vi "RSZVB Add Limit Line Segment.vi"(0 "VISA session":refnum<visa-resource-name>, 1 "Stop Stimulus (0.0)":dbl format="%^.3e", 2 "Stop Response (0.0)":dbl format="%^.3e", 5 "Channel (Trace) (1)":i32=1, 7 "Segment (1)":i32=1, 9 "Type (1: Upper)":i32(ring)=1 items=["Off", "Upper", "Lower"], 11 "error in (no error)":errorcluster {"code" format="%.0x"}, 12 "Start Response (0.0)":dbl format="%^.3e", 13 "Start Stimulus (0.0)":dbl format="%^.3e") -> (4 "dup VISA session":refnum<visa-resource-name>, 15 "error out":errorcluster {"code" format="%.0x"})   [LabVIEW 2011]
doc: "This VI adds a new segment to the limit line list. In each segment the limit line is defined as a straight line connecting two points.\n\nNote(s):\n\nThis VI does not overwrite existing limit line segments. The defined segment is appended to the segment list as new segment.\n\nRemote-control command(s):\nCALCulate<Ch/Tr>:LIMit:DATA <type>, <start_stim>, <stop_stim>, <start_resp>, <stop_resp>"
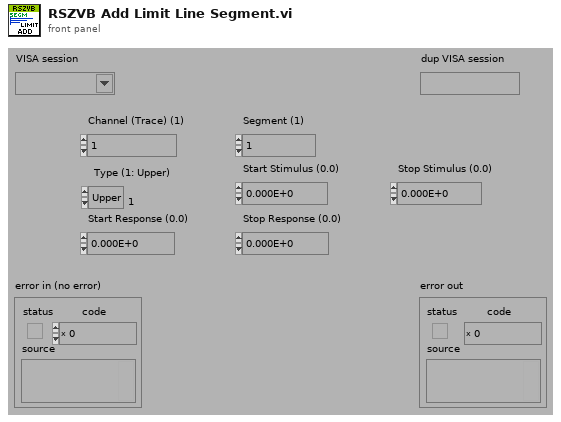
[diagram p1: front panel]
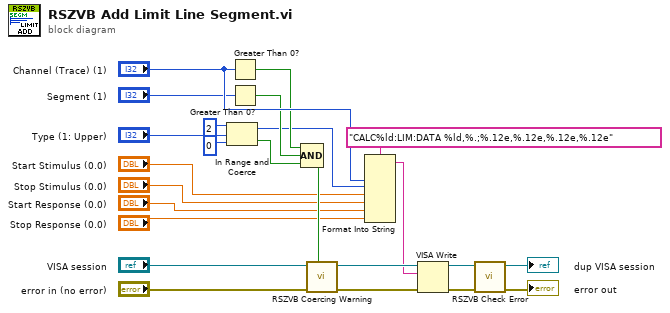
[diagram p0: block diagram]
diagram:
  n1 = In Range and Coerce(upper limit=2, x="Type (1: Upper)", lower limit=0) -> (coerced(x)=w2:i32, In Range?=w17:bool)
  n2 = Greater Than 0?(x="Channel (Trace) (1)") -> (x > 0?=w4:bool)
  n3 = Greater Than 0?(x="Segment (1)") -> (x > 0?=w3:bool)
  n4 = Compound Arithmetic op=AND(w4, w3, w17) -> (w16:bool)
  n5 = call "RSZVB Coercing Warning.vi"("In Range?"=w16, "error in (no error)"="error in (no error)", "VISA session"="VISA session") -> ("error out"=w23:errorcluster, "dup VISA session"=w24:refnum<visa-resource-name>)  [unwired: 7 in]
  n6 = Format Into String(format string="CALC%ld:LIM:DATA %ld,%.;%.12e,%.12e,%.12e,%.12e", "Channel (Trace) (1)", w2, "Start Stimulus (0.0)", "Stop Stimulus (0.0)", "Start Response (0.0)", "Stop Response (0.0)") -> (resulting string=w15:string)  [unwired: 2 in, 1 out]
  n7 = VISA Write(VISA resource name=w24, write buffer=w15, error in (no error)=w23) -> (VISA resource name out=w21:refnum<visa-resource-name>, error out=w22:errorcluster)  [unwired: 1 out]
  n8 = call "RSZVB Check Error.vi"("error in (no error)"=w22, "VISA session"=w21) -> ("error out"=→"error out":errorcluster, "dup VISA session"=→"dup VISA session":refnum<visa-resource-name>)  [unwired: 8 in]
